vi "Spont7.vi"() -> ()   [LabVIEW 2014]
uses:
  <vilib>/Utility/file.llb/Write To Spreadsheet File (DBL).vi
panel:
  out "Identification":string
  out "Running":bool caption="C867_Multiaxis_Configuration_Setup.vi is running"
  out "Position":dbl[](array[numeric]) format="%.6f"
  in  "PI Stage Error":errorcluster
  out "GndNum":dbl
  out "Current Set":u32=24
  in  "time zero":dbl
  in  "Number of ground/series":dbl
  in  "Time points (fs)":dbl[](array[numeric])
  in  "Number of Series":dbl
  in  "take series":bool
  out "Status":string="Shutter Closed"
  in  "Shutter Position":bool
  in  "width":dbl=100.0
  in  "bottom row":dbl
  out "delta_counts":dbl=5.100000000000023
  out "cursor y":dbl=598.3
  out "Intensity Graph":u16[][](graph)
  in  "focus":bool
  in  "Filename":string="test"
  in  "SetPath":bool
  in  "Path":string="C:\\data"
  in  "Multi Acquire":bool
  in  "Number of acquisitions":dbl=10.0 format="%.3f"
  in  "Acquire":bool
  out "Temperature":dbl=-75.0
  in  "stop":bool
  in  "Save?":bool
  out "Waveform Graph":dbl[](graph)=[588.6, 596.72, 595.34, 596.64, 595.2, 596.1, 597.16, 596.12, 597.8, 597.66, 595.06, 597.86, 598.22, 596.64, 596.76, 597.44, 597.16, 596.86, 598.62, 597.82, 597.82, 598.04, 596.38, 597.32, 598.0, 596.96, 597.12, 596.68, 597.72, 595.7, 598.18, 596.84, 596.3, 596.74, 598.34, 595.84, 597.76, 597.96, 596.3, 597.2, 596.78, 595.68, 597.16, 597.9, 596.24, 596.52, 597.42, 596.5, 596.02, 596.42, 596.72, 595.96, 596.42, 596.8, 597.3, 594.68, 597.84, 596.16, 596.06, 595.2, 595.82, 595.88, 596.94, 596.26, 596.28, 595.88, 595.68, 596.14, 596.9, 597.08, 597.12, 596.2, 595.18, 595.26, 595.72, 596.18, 595.52, 595.84, 595.86, 596.56, 595.58, 596.64, 595.9, 596.54, 595.7, 595.56, 596.3, 596.8, 595.74, 596.68, 595.48, 596.96, 596.12, 595.02, 596.08, 595.96, 596.34, 596.14, 595.98, 595.84, 596.5, 595.88, 596.6, 595.96, 596.86, 596.28, 596.22, 595.8, 595.46, 596.18, 596.32, 596.0, 596.12, 596.22, 595.82, 595.76, 597.1, 596.46, 596.86, 596.48, 595.66, 595.94, 596.38, 595.46, 596.12, 596.36, 596.46, 596.7, 596.32, 596.84, 594.96, 595.22, 596.56, 596.52, 595.72, 596.22, 596.22, 596.38, 596.8, 595.52, 596.92, 597.12, 595.92, 596.18, 596.5, 597.3, 596.4, 596.46, 596.28, 597.04, 596.42, 595.84, 597.12, 596.66, 596.2, 597.02, 596.22, 596.12, 596.78, 595.68, 596.02, 595.36, 596.5, 596.9, 595.76, 595.12, 596.72, 597.54, 596.32, 596.76, 597.82, 597.52, 595.5, 595.88, 597.38, 596.3, 597.58, 595.42, 597.12, 597.58, 596.98, 597.44, 595.9, 596.58, 596.78, 597.04, 597.2, 596.06, 596.58, 597.08, 598.68, 596.32, 597.3, 597.28, 597.26, 595.9, 597.3, 597.98, 598.08, 598.16, 596.42, 597.82, 596.88, 597.34, 598.22, 598.38, 598.34, 597.66, 596.98, 597.18, 597.18, 597.7, 598.3, 597.3, 596.28, 597.0, 598.0, 598.42, 597.96, 596.32, 598.76, 597.32, 598.08, 598.1, 598.14, 598.06, 597.46, 598.08, 597.1, 597.88, 597.76, 598.74, 598.2, 598.54, 598.26, 596.74, 597.4, 597.82, 597.4, 597.64, 598.78, 597.84, 598.28, 596.68, 597.44, 598.66, 597.94, 598.2, 598.82, 598.28, 598.5, 597.86, 599.04, 597.96, 597.22, 598.38, 597.72, 598.18, 598.58, 598.44, 598.64, 598.98, 597.94, 598.84, 599.02, 598.76, 599.08, 599.0, 598.78, 597.5, 599.4, 598.52, 599.9, 597.04, 598.76, 598.3, 598.88, 599.76, 598.54, 599.92, 597.88, 598.42, 599.8, 599.8, 599.24, 598.58, 598.76, 597.02, 599.76, 599.84, 598.98, 599.5, 599.58, 599.46, 598.08, 599.3, 598.56, 598.74, 598.98, 598.74, 599.04, 599.18, 599.08, 598.64, 598.88, 599.04, 599.3, 598.54, 600.1, 599.12, 600.02, 599.32, 599.74, 600.04, 599.44, 598.96, 599.82, 601.1, 600.46, 599.48, 601.04, 599.16, 601.68, 600.5, 599.06, 599.0, 600.26, 600.54, 599.88, 599.62, 600.82, 601.56, 600.38, 600.6, 601.6, 599.1, 601.64, 600.56, 600.8, 601.94, 600.82, 599.68, 602.12, 602.36, 600.5, 601.56, 601.62, 601.04, 601.0, 602.0, 600.66, 601.34, 601.52, 600.86, 601.7, 600.28, 602.32, 602.78, 601.06, 600.34, 602.7, 602.52, 602.5, 601.3, 603.24, 601.06, 603.72, 603.78, 602.12, 601.68, 603.34, 602.0, 602.46, 602.64, 603.3, 601.6, 603.18, 603.1, 602.74, 602.32, 602.3, 603.38, 602.02, 602.82, 604.16, 603.64, 603.32, 603.84, 604.06, 603.82, 603.56, 602.68, 605.1, 602.58, 603.42, 603.36, 603.76, 602.68, 602.68, 602.22, 604.3, 602.44, 603.86, 603.74, 603.18, 603.32, 603.98, 604.28, 604.5, 602.92, 602.02, 604.08, 604.02, 604.02, 603.46, 603.42, 604.62, 602.96, 603.08, 604.44, 604.38, 603.66, 604.1, 603.98, 603.26, 603.46, 603.96, 604.54, 603.78, 603.98, 604.08, 604.18, 604.32, 605.34, 603.34, 605.42, 603.56, 604.22, 604.34, 604.32, 603.9, 603.66, 604.04, 605.02, 604.48, 604.16, 603.02, 603.8, 604.44, 604.66, 604.68, 604.12, 605.02, 604.86, 605.3, 604.54, 605.84, 604.78, 605.76, 604.86, 604.44, 605.16, 605.16, 604.86, 604.06, 605.46, 604.4, 603.62, 606.52, 606.38, 604.6, 605.34, 605.34, 604.98, 603.98, 605.5, 605.6, 604.54, 604.48, 604.3, 606.24, 605.36, 605.48, 605.36, 606.14, 605.26, 603.84, 604.94, 605.2, 605.16, 606.34, 604.56, 605.56, 605.74, 605.32, 605.34, 606.02, 607.14, 606.36, 605.08, 605.38, 606.54, 606.18, 607.14, 606.44, 606.22, 606.9, 606.66, 606.82, 606.76, 606.52, 606.24, 607.18, 606.6, 607.16, 609.14, 606.86, 606.68, 608.42, 606.66, 608.94, 608.54, 608.66, 608.4, 608.54, 608.54, 608.22, 608.26, 608.86, 608.4, 607.54, 607.48, 608.34, 610.3, 608.64, 607.96, 608.46, 609.12, 609.04, 607.74, 607.94, 609.82, 608.42, 609.24, 609.6, 608.64, 607.96, 608.92, 609.96, 609.78, 609.4, 608.54, 608.72, 607.38, 608.34, 609.22, 608.02, 608.38, 609.44, 608.12, 609.24, 609.06, 607.92, 609.1, 607.34, 609.76, 609.0, 609.04, 608.88, 607.82, 607.98, 608.34, 608.52, 609.72, 607.86, 608.1, 608.16, 607.1, 608.88, 606.4, 608.84, 608.48, 607.32, 608.34, 607.24, 608.02, 607.8, 608.04, 607.02, 608.8, 607.88, 608.4, 607.34, 607.66, 606.8, 607.2, 607.66, 608.94, 607.64, 608.6, 608.32, 607.64, 608.2, 608.02, 608.74, 607.9, 609.06, 606.98, 607.78, 607.6, 608.42, 607.68, 609.02, 608.2, 608.96, 607.76, 607.78, 608.84, 608.14, 609.02, 607.94, 608.8, 608.26, 608.9, 607.42, 608.9, 608.52, 607.1, 608.34, 608.44, 608.88, 608.28, 607.54, 607.88, 607.48, 608.28, 608.74, 608.64, 607.36, 608.72, 608.18, 608.5, 608.26, 609.14, 608.68, 608.34, 608.52, 608.24, 609.26, 609.5, 609.1, 607.4, 609.28, 609.72, 609.9, 609.22, 609.72, 609.66, 608.96, 609.84, 610.84, 610.26, 609.92, 609.36, 609.5, 609.14, 609.68, 609.52, 609.3, 608.82, 611.08, 610.52, 610.36, 610.02, 609.26, 609.7, 610.56, 609.24, 610.14, 609.78, 609.4, 611.1, 611.3, 611.64, 612.6, 610.7, 613.46, 611.62, 612.18, 610.72, 613.36, 612.92, 613.4, 612.44, 613.96, 612.2, 613.78, 615.38, 613.92, 613.36, 613.88, 615.7, 613.32, 613.66, 615.56, 615.4, 615.74, 616.56, 617.68, 614.58, 615.08, 616.86, 614.2, 615.56, 616.52, 616.36, 615.24, 616.04, 615.78, 615.56, 614.72, 616.18, 614.7, 614.36, 613.78, 614.8, 613.68, 614.04, 614.34, 613.14, 613.64, 613.64, 614.42, 612.28, 613.78, 612.32, 613.28, 611.98, 613.0, 612.32, 611.54, 612.3, 612.14, 610.24, 611.56, 611.84, 609.42, 610.02, 608.86, 609.02, 608.0, 609.18, 608.92, 608.78, 608.16, 608.16, 607.16, 607.6, 605.94, 607.6, 607.18, 607.04, 607.18, 605.5, 607.02, 605.26, 604.78, 606.2, 605.3, 604.52, 604.9, 604.58, 603.74, 604.46, 605.02, 603.8, 604.58, 603.5, 603.18, 603.26, 603.48, 603.56, 604.36, 602.92, 602.44, 603.58, 604.18, 603.16, 602.2, 603.7, 603.12, 602.68, 601.74, 602.14, 602.48, 602.62, 602.0, 602.22, 602.06, 600.94, 601.92, 601.28, 602.22, 601.72, 601.44, 602.04, 603.22, 601.52, 601.36, 602.06, 601.96, 602.14, 601.68, 601.28, 602.46, 601.56, 601.44, 602.1, 602.1, 601.8, 603.02, 601.12, 599.86, 601.56, 600.46, 601.28, 601.18, 600.58, 599.68, 600.74, 600.74, 601.66, 600.72, 600.6, 602.3, 599.66, 601.5, 602.32, 601.38, 600.18, 600.76, 601.32, 599.64, 601.16, 599.82, 600.52, 600.66, 601.66, 600.36, 600.18, 599.8, 601.42, 601.12, 599.68, 600.6, 600.42, 599.92, 600.98, 600.56, 599.54, 600.46, 601.52, 601.1, 599.78, 600.84, 599.98, 600.6, 599.16, 599.74, 600.46, 600.42, 600.62, 599.84, 599.66, 600.98, 600.98, 600.94, 601.16, 602.18, 601.28, 600.56, 601.56, 600.94, 602.32, 600.34, 601.98, 602.02, 601.46, 602.86, 603.68, 603.04, 601.86, 602.02, 601.94, 602.36, 601.96, 602.14, 602.42, 603.9, 602.9, 602.66, 602.48, 603.4, 603.32, 601.5, 603.14, 601.3, 601.94, 603.14, 602.58, 601.6, 600.16, 602.08, 600.76, 599.68, 602.42, 601.32, 600.14, 600.22, 599.8, 600.3, 598.68, 599.82, 599.72, 599.24, 599.36, 599.64, 599.34, 598.94, 598.82, 598.82, 597.72, 599.52, 598.6, 598.18, 597.34, 598.04, 597.26, 598.3, 598.18, 597.88, 596.96, 598.36, 597.14, 597.7, 597.7, 598.32, 597.54, 598.62, 596.16, 598.24, 598.36, 596.74, 597.62, 597.46, 596.92, 597.18, 598.18, 597.04, 596.94, 596.78, 596.92, 597.72, 596.84, 596.98, 597.02, 597.44, 597.34, 597.98, 596.28, 598.24, 597.62, 596.52, 596.6, 597.32, 596.58, 597.78, 597.82, 596.64, 596.28, 597.64, 597.14, 597.4, 597.42, 597.6, 596.1, 597.04, 597.94, 597.38, 597.08, 597.4, 597.66, 596.64, 597.68, 597.6, 596.6, 598.68, 597.3, 596.06, 596.9, 596.22, 597.14, 596.6, 597.3, 596.32, 596.6, 596.8, 595.5, 597.28, 597.02, 596.42, 596.58, 595.22, 596.26, 597.54, 597.24, 597.04, 596.62, 597.18, 596.72, 596.56, 596.82, 596.96, 595.0, 595.9, 596.66, 596.98, 595.36, 595.84, 596.92, 596.84, 596.5, 598.1, 595.56, 596.7, 596.2, 596.66, 595.92, 597.0, 596.86, 595.82, 596.24, 596.7, 596.66, 596.36, 597.12, 597.48, 596.52, 598.24, 596.88, 596.66, 596.18, 597.32, 596.68, 596.6, 597.56, 597.46, 597.28, 596.44, 598.22, 596.78, 597.58, 596.9, 597.02, 597.7, 598.36, 597.7, 597.82, 597.6, 596.76, 598.34, 596.64, 597.76, 597.26, 597.26, 597.2, 598.16, 598.38, 596.48, 597.54, 598.78, 597.72, 597.6, 596.28, 597.92, 596.92, 597.46, 597.82, 597.7, 596.92, 598.0, 598.34, 598.0, 598.1, 596.42, 597.68, 597.0, 597.04, 598.34, 598.08, 598.16, 597.44, 596.68, 598.76, 598.98, 597.34, 598.54, 597.74, 598.16, 597.02, 597.82, 596.48, 599.84, 598.26, 599.96, 598.18, 598.06, 596.84, 597.94, 597.86, 597.82, 597.2, 597.74, 598.74, 598.66, 599.84, 599.12, 599.16, 598.22, 599.14, 598.3, 599.32, 599.28, 598.04, 599.02, 600.24, 598.9, 598.52, 600.26, 599.12, 599.52, 600.16, 598.7, 600.54, 600.4, 600.34, 599.94, 601.08, 601.94, 601.8, 601.84, 600.94, 602.66, 602.7, 603.24, 603.4, 603.48, 603.54, 604.46, 603.48, 604.86, 604.02, 605.42, 605.5, 605.6, 605.66, 606.92, 606.64, 607.8, 608.02, 606.8, 607.34, 608.3, 608.7, 609.58, 607.02, 608.78, 609.04, 608.58, 608.68, 607.9, 607.96, 608.04, 606.88, 607.1, 608.22, 606.34, 606.48, 605.72, 607.14, 607.1, 606.26, 605.84, 605.2, 606.94, 605.42, 605.78, 604.82, 604.0, 604.46, 604.06, 604.12, 604.18, 602.44, 602.64, 602.74, 602.96, 602.62, 602.58, 601.22, 601.08, 601.62, 601.8, 600.3, 600.86, 600.84, 601.36, 601.52, 600.26, 601.46, 601.82, 601.08, 601.38, 600.68, 601.24, 600.14, 600.86, 601.44, 601.02, 601.64, 600.2, 600.14, 600.08, 601.2, 600.78, 600.14, 600.7, 600.84, 600.46, 600.52, 601.54, 600.18, 601.48, 601.34, 600.8, 600.14, 600.98, 601.96, 601.24, 599.72, 601.54, 601.0, 601.22, 602.3, 601.8, 600.8, 602.04, 601.66, 602.18, 602.98, 601.9, 600.84, 601.02, 602.26, 602.6, 601.68, 602.74, 603.4, 603.34, 601.14, 603.26, 603.8, 602.5, 605.12, 607.2, 608.98, 613.54, 618.18, 624.58, 630.92, 637.18, 645.2, 652.4, 662.02, 675.08, 685.88, 712.56, 745.04, 764.62, 788.84, 800.84, 817.9, 850.88, 881.62, 935.36, 970.52, 991.22, 1024.2, 1039.16, 1063.5, 1047.88, 1030.98, 1037.14, 1049.92, 1025.08, 960.02, 939.14, 920.52, 907.38, 895.3, 884.3, 860.94, 811.92, 782.22, 752.82, 733.08, 720.42, 706.32, 693.9, 683.38, 676.24, 667.8, 659.5, 652.08, 648.94, 646.08, 642.08, 637.86, 633.48, 631.2, 628.9, 626.92, 625.0, 622.5, 622.22, 619.52, 621.44, 618.92, 619.38, 619.44]
  in  "Exposure Time (s)":dbl=20.0 format="%.3f"
  out "error out":errorcluster
  in  "error in (no error)":errorcluster
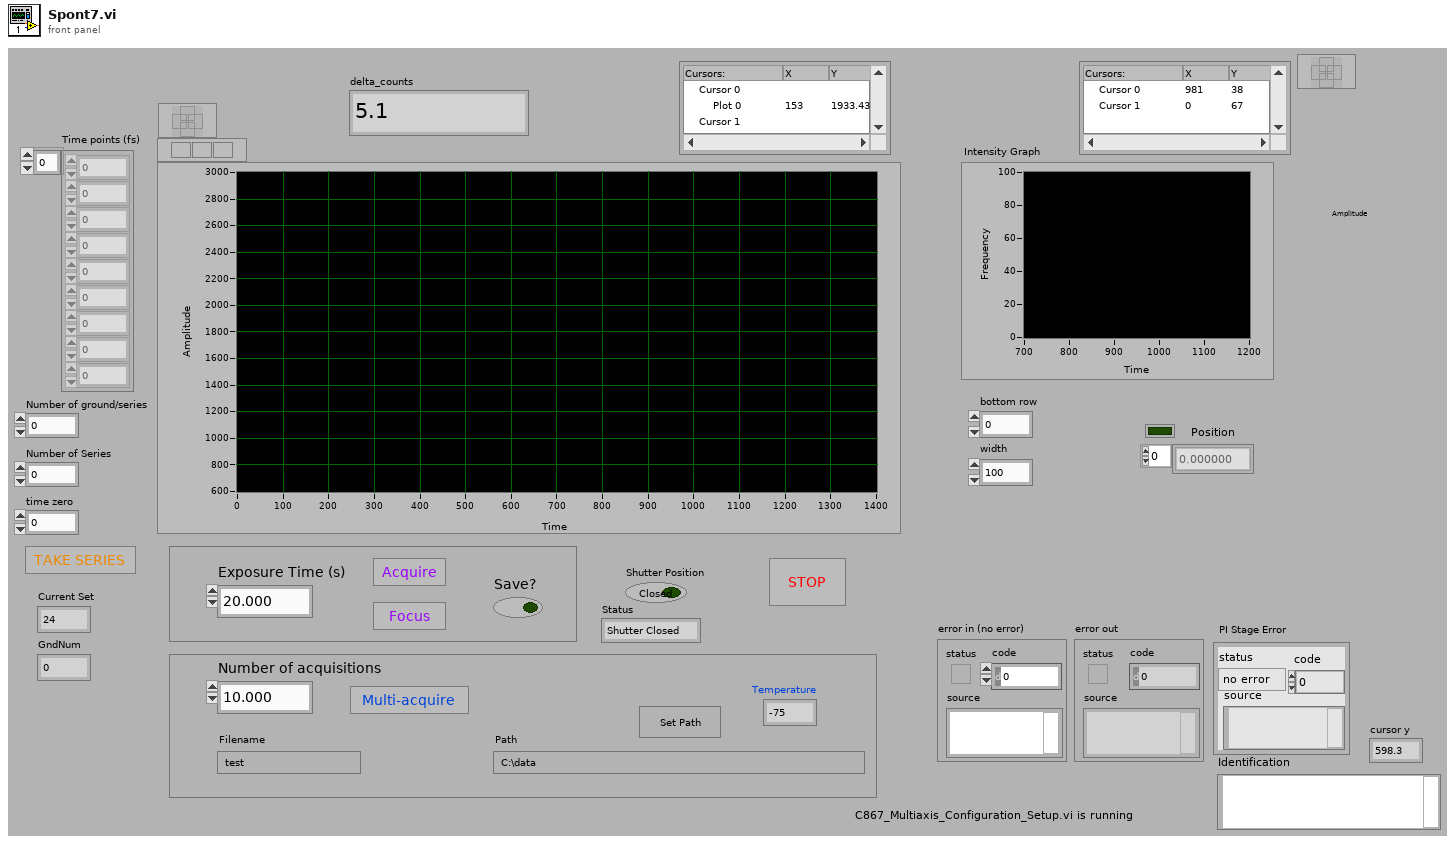
[diagram p1: front panel]
types:
  T1 = cluster{"Camera Handle":u32, "File Handle":u32, "Image Handle":u32}
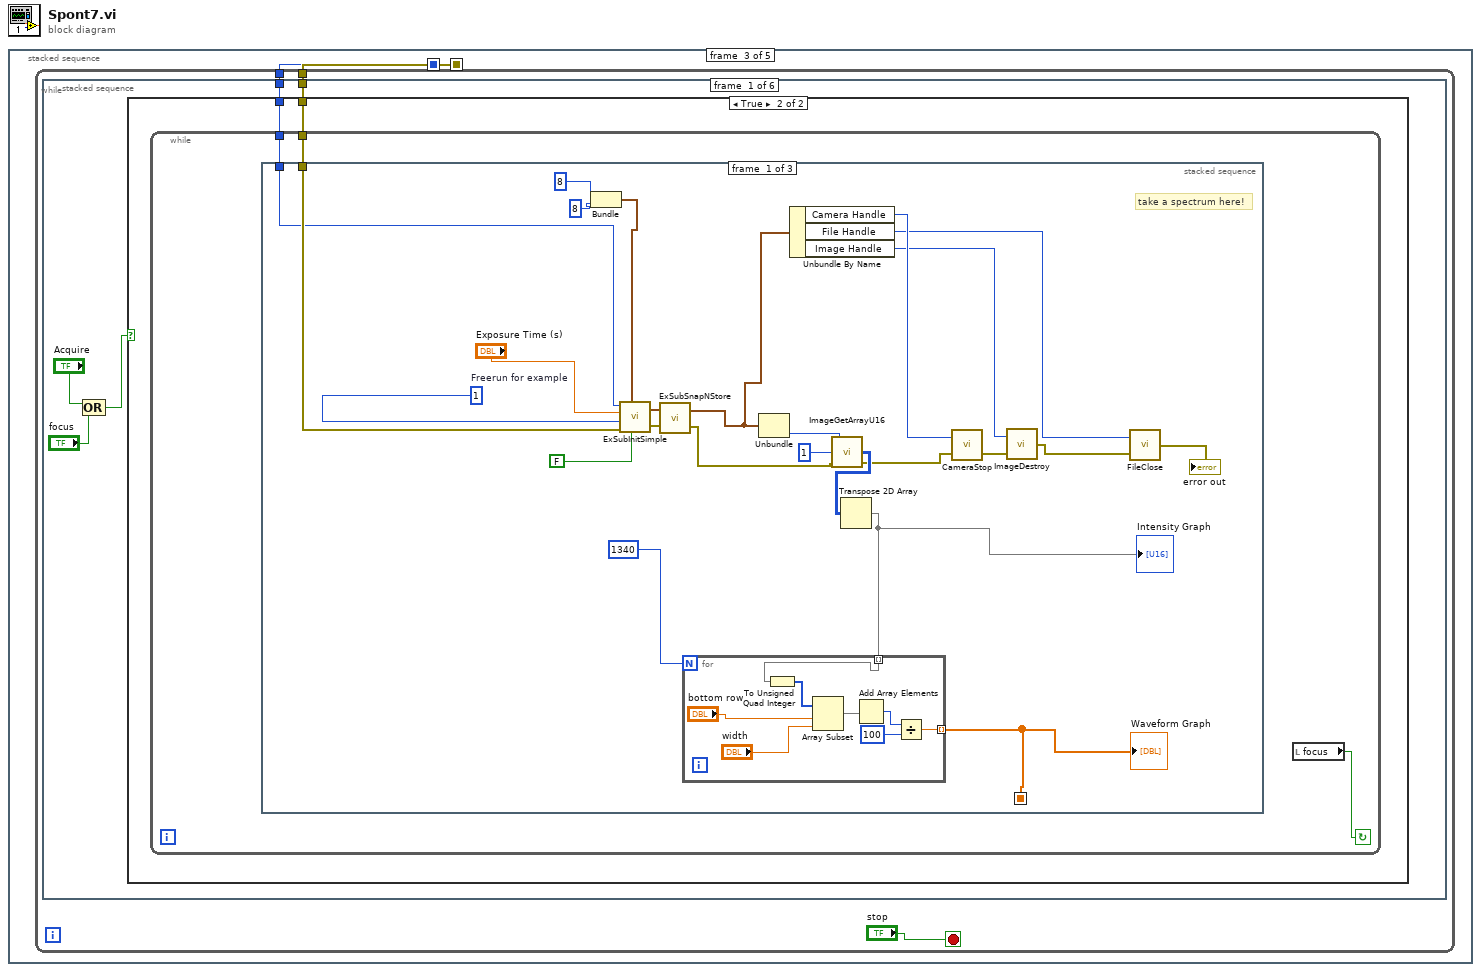
[diagram p0: block diagram]
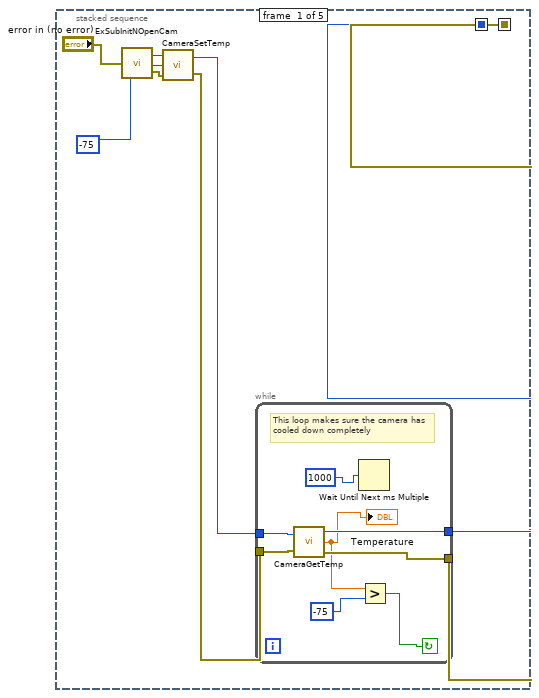
[diagram p2: hidden frame]
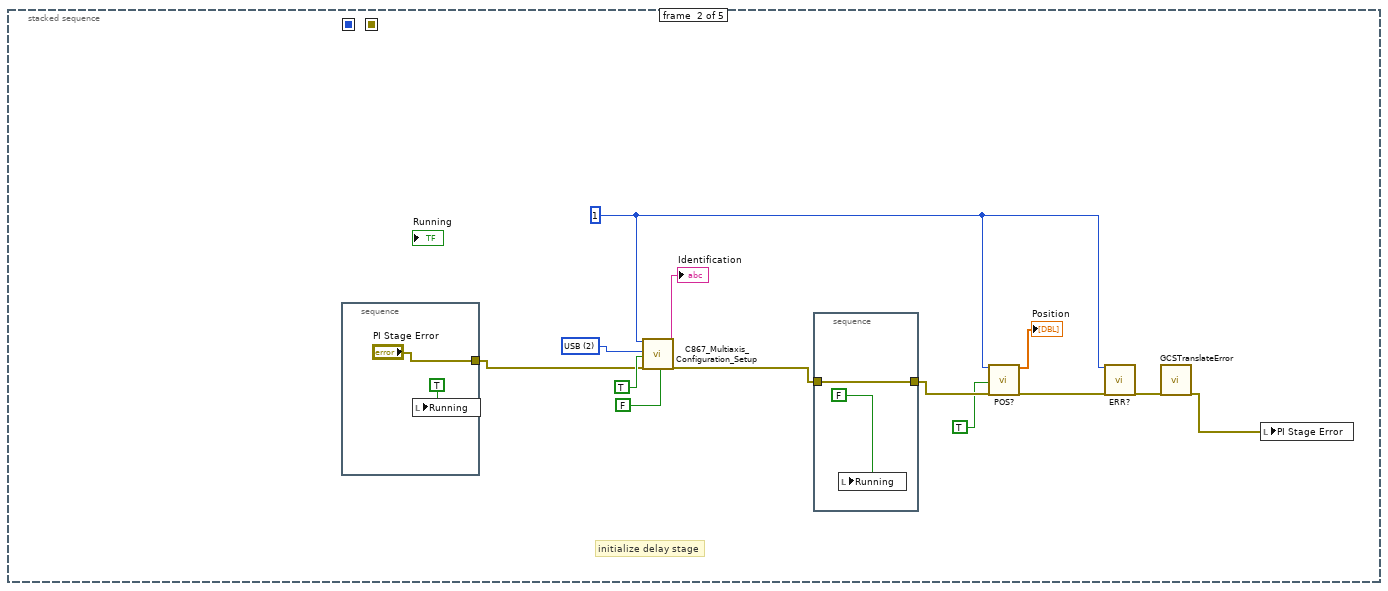
[diagram p3: hidden frame]
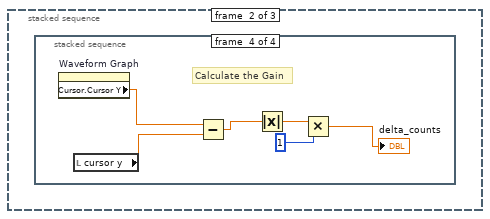
[diagram p5: hidden frame]
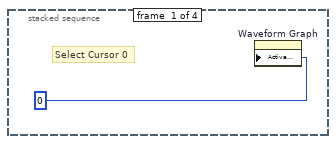
[diagram p6: hidden frame]
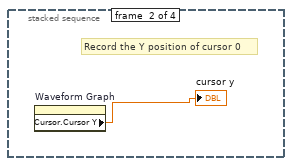
[diagram p7: hidden frame]
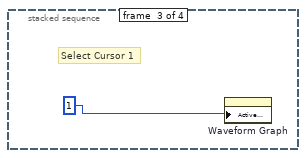
[diagram p8: hidden frame]
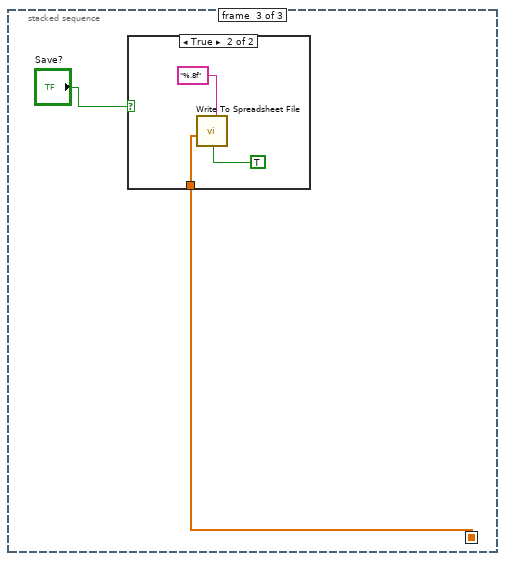
[diagram p9: hidden frame]
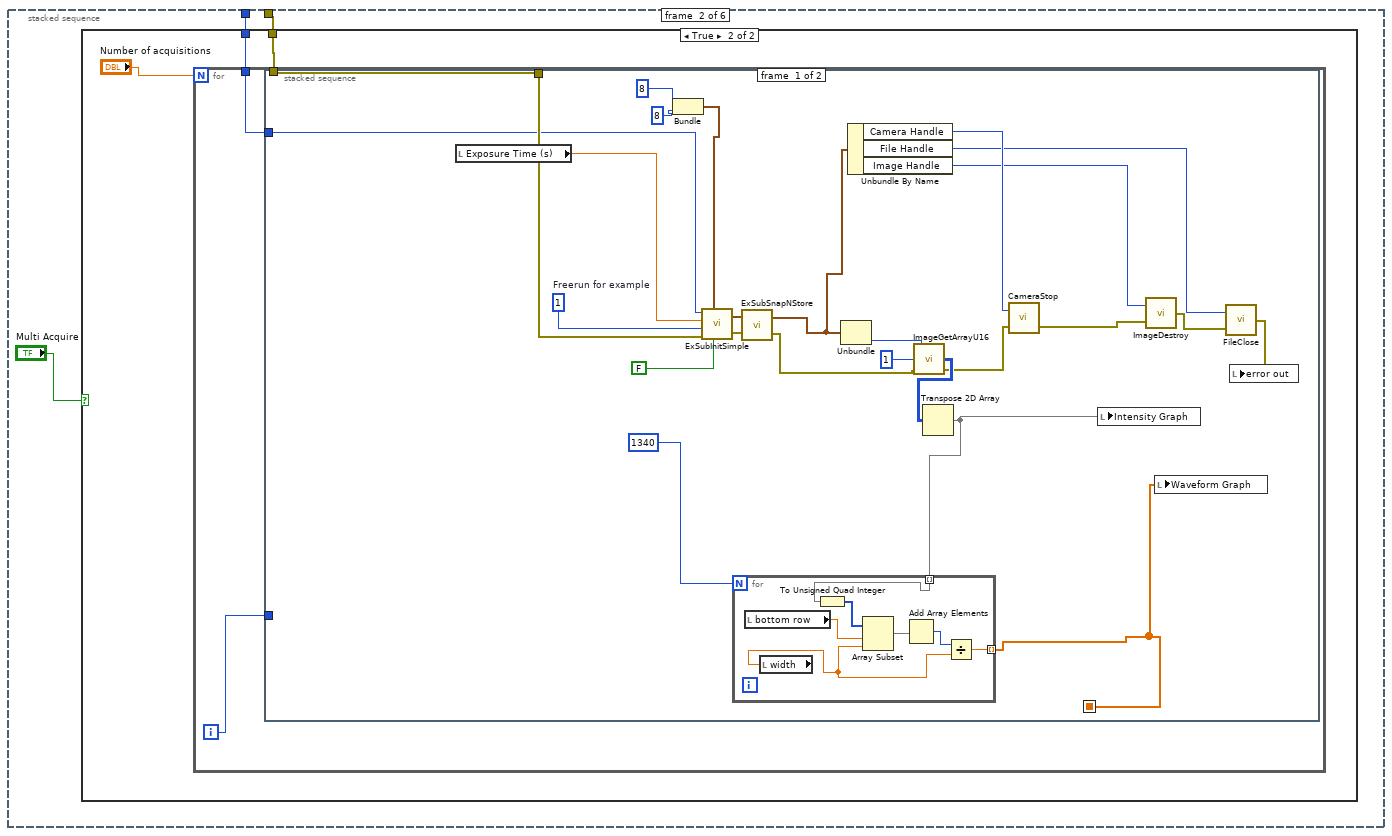
[diagram p11: hidden frame]
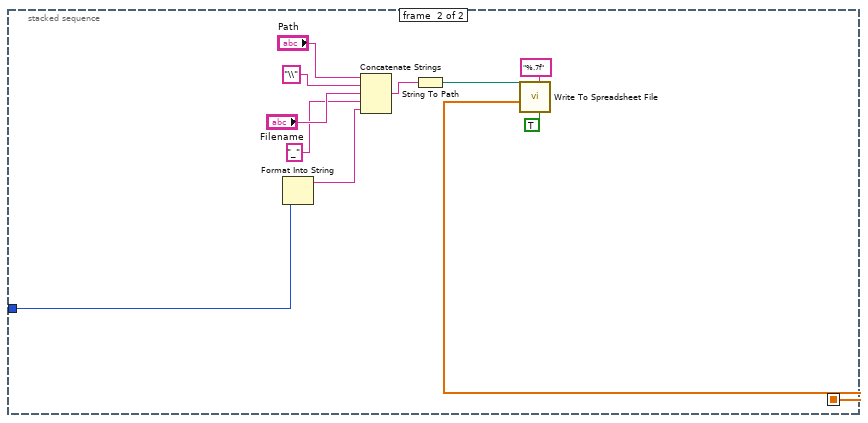
[diagram p13: hidden frame]
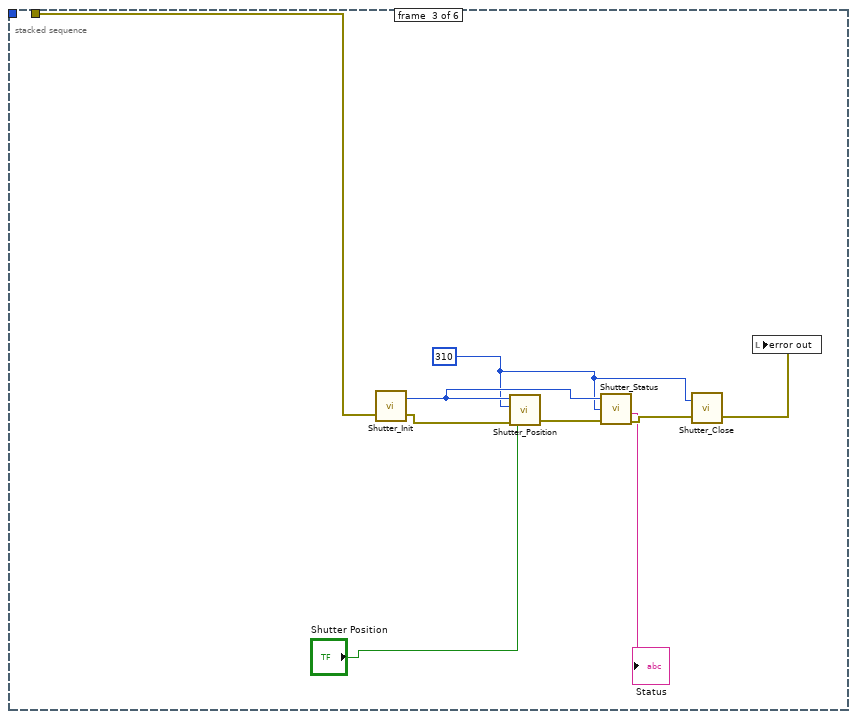
[diagram p14: hidden frame]
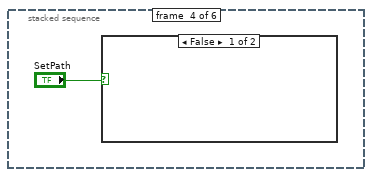
[diagram p15: hidden frame]
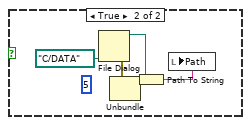
[diagram p16: hidden frame]
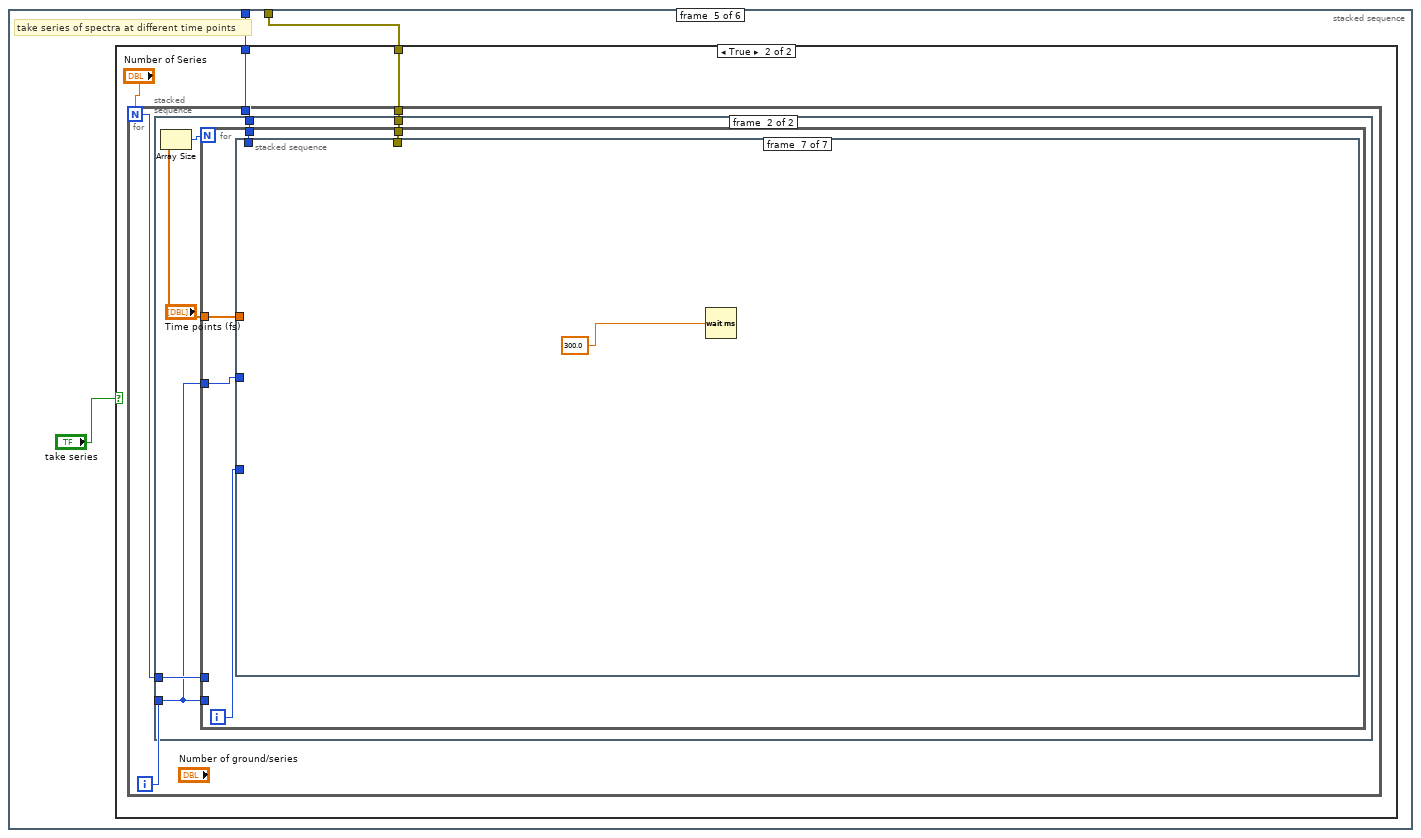
[diagram p17: hidden frame]
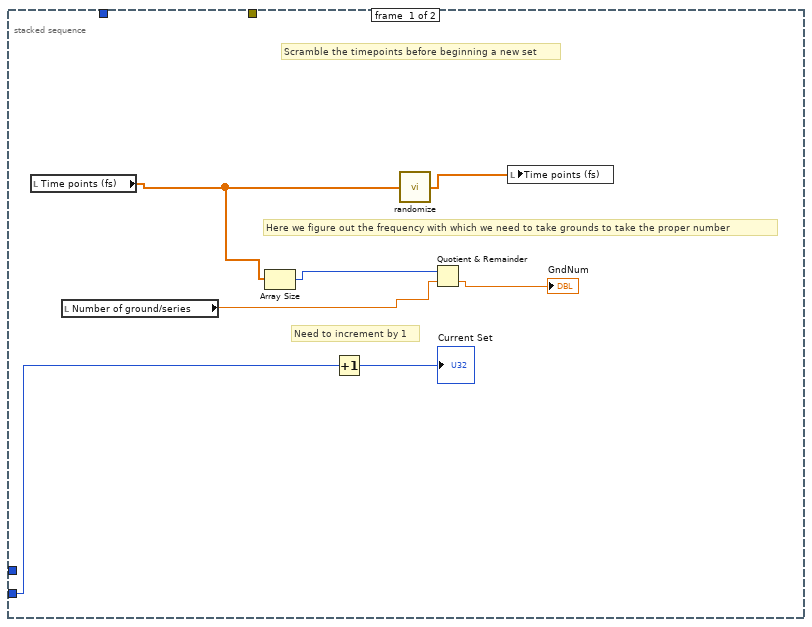
[diagram p19: hidden frame]
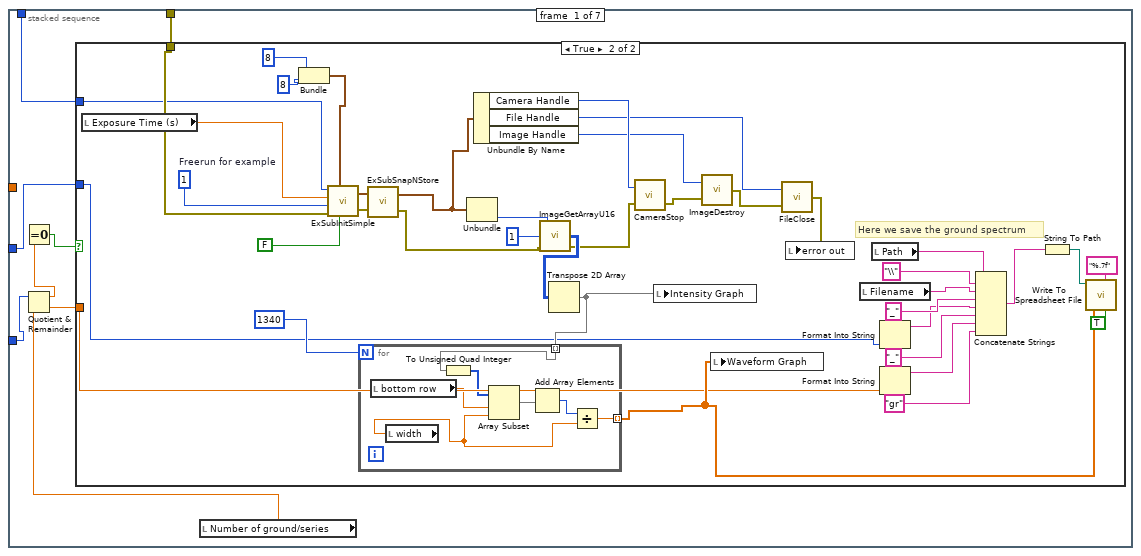
[diagram p20: hidden frame]
diagram:
  n1 = stacked-sequence {
    seq-local: [w2 _ _ _ _] -> [_ _ w35 _ w325]
    seq-local: [w1 _ _ _ _] -> [_ _ w34 _ w326]
    frame #0 {
      n2 = call "ExSubInitNOpenCam.vi"("error in (no error)"="error in (no error)") -> ("Camera Handle"=w5:u32, "error out"=w7:errorcluster)
      n3 = call <userlib>:"CameraSetTemp.vi"("error in (no error)"=w7, "Temperature"=-75, "Camera Handle"=w5) -> ("error out"=w3:errorcluster, "Camera Handle"=w4:u32)
      n4 = while {
        tunnel: w3 -> [w15]
        tunnel: [w14] -> w2
        tunnel: w4 -> [w13]
        tunnel: [w12] -> w1
        stop <- w10 continue-if-true
        # "This loop makes sure the camera has cooled down completely"
        n5 = call <userlib>:"CameraGetTemp.vi"("Camera Handle"=w13, "error in (no error)"=w15) -> ("Camera Handle"=w12:u32, "Temperature"=w9:dbl, "error out"=w14:errorcluster)
        "Temperature" <- w9
        n6 = Wait Until Next ms Multiple(millisecond multiple=1000 ("ADC Gain")) -> ()  [unwired: 1 out]
        n7 = Greater?(x=w9, y=-75) -> (0:w10:bool)
      }
    }
    frame #1 {
      w20 = 1 ("System no.")
      w29 = u16 2 items=["RS232", "RS232 DaisyChain", "USB"] ("Interface")
      # "initialize delay stage"
      n8 = stacked-sequence {
        tunnel: ["PI Stage Error"] -> w26
        frame #0 {
          n9 = local write "Running"(TRUE ("Running")) -> ()
        }
      }
      n10 = call "C867_Multiaxis_Configuration_Setup.vi"("System no."=w20, "Interface"=w29, "All axes?"=TRUE, "error in"=w26, "Switch servo on?"=FALSE ("Use dialog to define\nconnected stages?")) -> ("Identification"=→"Identification":string, "error out"=w25:errorcluster)  [unwired: 8 in, 5 out]
      n11 = stacked-sequence {
        tunnel: w25 -> [w31]
        tunnel: [w31] -> w23
        frame #0 {
          n12 = local write "Running"(FALSE ("Running")) -> ()
        }
      }
      n13 = call "POS?.vi"("System no."=w20, "All axes?"=TRUE, "error in"=w23) -> ("Position"=→"Position":dbl[], "error out"=w21:errorcluster)  [unwired: 15 in]
      n14 = call "ERR?.vi"("System no."=w20, "error in"=w21) -> ("error out"=w19:errorcluster)  [unwired: 16 in, 1 out]
      n15 = call "GCSTranslateError.vi"("error in"=w19) -> ("error out"=w17:errorcluster)  [unwired: 16 in, 2 out]
      n16 = local write "PI Stage Error"(w17) -> ()
    }
    frame #2 {
      n17 = while {
        tunnel: w35 -> [w37]
        tunnel: w34 -> [w36]
        stop <- "stop" stop-if-true
        n18 = stacked-sequence {
          tunnel: w37 -> [w43 w97 w149 _ w163 _]
          tunnel: w36 -> [w42 w96 _ _ w162 _]
          frame #0 {
            n19 = Compound Arithmetic op=OR("Acquire", "focus") -> (w39:bool)
            n20 = case shown="True" w39 {
              tunnel: w43 -> [_ w45]
              tunnel: w42 -> [_ w44]
              frame False {
              }
              frame True {
                n21 = while {
                  tunnel: w45 -> [w48]
                  tunnel: w44 -> [w47]
                  stop <- w46 continue-if-true
                  n22 = stacked-sequence {
                    seq-local: [w60 _ _] -> [_ _ w91]
                    tunnel: w48 -> [w59 _ _]
                    tunnel: w47 -> [w58 _ _]
                    frame #0 {
                      w71 = 1  # Freerun for example
                      # "take a spectrum here!"
                      n23 = Bundle(8, 8) -> (w69:cluster{i32, i32})  [unwired: 1 in]
                      n24 = call "ExSubInitSimple.vi"("Intensifier"=FALSE, "Shutter Comp"=w69, "error in (no error)"=w59, "Triggering mode"=w71, "Exposure"="Exposure Time (s)", "Camera Handle"=w58) -> ("error out"=w68:errorcluster, "Handles"=w67:cluster{"Camera":u32, "File":u32, "Image":u32})
                      n25 = call "ExSubSnapNStore.vi"("error in (no error)"=w68, "Handle Cluster"=w67) -> ("error out"=w63:errorcluster, "Handle Cluster Out"=w57:T1)
                      n26 = Unbundle(w57) -> ("Image Handle"=w64:u32)  [unwired: 2 out]
                      n27 = Unbundle By Name(w57) -> ("Camera Handle"=w56:u32, "File Handle"=w55:u32, "Image Handle"=w52:u32)
                      n28 = call <userlib>:"ImageGetArrayU16.vi"("error in"=w63, "Z position"=1, "Image Handle"=w64) -> ("error out"=w54:errorcluster, "Array uint 16"=w62:u16[][])  [unwired: 1 out]
                      n29 = Transpose 2D Array(2D array=w62) -> (transposed array=w49:u16[][])
                      "Intensity Graph" <- w49
                      n30 = for {
                        N: 1340 -> [_]
                        tunnel: w49 -> [w78] mode=indexing
                        tunnel: [w80] -> w60 mode=indexing
                        n31 = To Unsigned Quad Integer(1:w78) -> (0:w77:u64[])
                        n32 = Array Subset(array=w77, index="bottom row", length="width") -> (w79:u64[])
                        n33 = Add Array Elements(numeric array=w79) -> (sum=w81:u64)
                        n34 = Divide(x=w81, y=u64 100) -> (x/y=w80:dbl)
                      }
                      "Waveform Graph" <- w60
                      n35 = call <userlib>:"CameraStop.vi"("error in"=w54, "Camera Handle"=w56) -> ("error out"=w51:errorcluster)  [unwired: 1 out]
                      n36 = call <userlib>:"ImageDestroy.vi"("error in"=w51, "Data handle"=w52) -> ("error out"=w50:errorcluster)
                      n37 = call <userlib>:"FileClose.vi"("error in"=w50, "File Handle"=w55) -> ("error out"=→"error out":errorcluster)
                    }
                    frame #1 {
                      n38 = stacked-sequence {
                        frame #0 {
                          # "Select Cursor 0"
                          n39 = property on="Waveform Graph" class="WFGraph (strict)"("Active Cursor"=0) -> ()  [unwired: 2 in, 2 out]
                        }
                        frame #1 {
                          # "Record the Y position of cursor 0"
                          n40 = property on="Waveform Graph" class="WFGraph (strict)"() -> ("Cursor.Cursor Y"=→"cursor y":dbl)  [unwired: 2 in, 2 out]
                        }
                        frame #2 {
                          # "Select Cursor 1"
                          n41 = property on="Waveform Graph" class="WFGraph (strict)"("Active Cursor"=1) -> ()  [unwired: 2 in, 2 out]
                        }
                        frame #3 {
                          # "Calculate the Gain"
                          n42 = property on="Waveform Graph" class="WFGraph (strict)"() -> ("Cursor.Cursor Y"=w85:dbl)  [unwired: 2 in, 2 out]
                          n43 = local read "cursor y"() -> (w90:dbl)
                          n44 = Subtract(x=w85, y=w90) -> (x-y=w87:dbl)
                          n45 = Absolute Value(x=w87) -> (abs(x)=w89:dbl)
                          n46 = Multiply(x=w89, y=1) -> (x*y=→"delta_counts":dbl)
                        }
                      }
                    }
                    frame #2 {
                      n47 = case shown="True" "Save?" {
                        tunnel: w91 -> [_ w94]
                        frame False {
                        }
                        frame True {
                          n48 = call-poly <vilib>:"Write To Spreadsheet File.vi"("transpose? (no:F)"=TRUE, "format (%.3f)"="%.8f", "1D data"=w94) -> ()  [unwired: 5 in, 1 out]
                        }
                      }
                    }
                  }
                  n49 = local read "focus"() -> (w46:bool)
                }
              }
            }
          }
          frame #1 {
            n50 = case shown="True" "Multi Acquire" {
              tunnel: w97 -> [_ w100]
              tunnel: w96 -> [_ w99]
              frame False {
              }
              frame True {
                n51 = for {
                  N: "Number of acquisitions" -> [_]
                  tunnel: w100 -> [w103]
                  tunnel: w99 -> [w102]
                  i -> [w104]
                  n52 = stacked-sequence {
                    seq-local: [w106 _] -> [_ w137]
                    tunnel: w104 -> [_ w147]
                    tunnel: w103 -> [w118 _]
                    tunnel: w102 -> [w117 _]
                    frame #0 {
                      w127 = 1  # Freerun for example
                      n53 = local read "Exposure Time (s)"() -> (w116:dbl)
                      n54 = Bundle(8, 8) -> (w126:cluster{i32, i32})  [unwired: 1 in]
                      n55 = call "ExSubInitSimple.vi"("Intensifier"=FALSE, "Shutter Comp"=w126, "error in (no error)"=w118, "Triggering mode"=w127, "Exposure"=w116, "Camera Handle"=w117) -> ("error out"=w125:errorcluster, "Handles"=w124:cluster{"Camera":u32, "File":u32, "Image":u32})
                      n56 = call "ExSubSnapNStore.vi"("error in (no error)"=w125, "Handle Cluster"=w124) -> ("error out"=w120:errorcluster, "Handle Cluster Out"=w113:T1)
                      n57 = Unbundle(w113) -> ("Image Handle"=w121:u32)  [unwired: 2 out]
                      n58 = Unbundle By Name(w113) -> ("Camera Handle"=w115:u32, "File Handle"=w114:u32, "Image Handle"=w109:u32)
                      n59 = call <userlib>:"ImageGetArrayU16.vi"("error in"=w120, "Z position"=1, "Image Handle"=w121) -> ("error out"=w112:errorcluster, "Array uint 16"=w119:u16[][])  [unwired: 1 out]
                      n60 = Transpose 2D Array(2D array=w119) -> (transposed array=w105:u16[][])
                      n61 = for {
                        N: 1340 -> [_]
                        tunnel: w105 -> [w133] mode=indexing
                        tunnel: [w135] -> w106 mode=indexing
                        n62 = local read "bottom row"() -> (w131:dbl)
                        n63 = local read "width"() -> (w130:dbl)
                        n64 = To Unsigned Quad Integer(1:w133) -> (0:w132:u64[])
                        n65 = Array Subset(array=w132, index=w131, length=w130) -> (w134:u64[])
                        n66 = Add Array Elements(numeric array=w134) -> (sum=w136:u64)
                        n67 = Divide(x=w136, y=w130) -> (x/y=w135:dbl)
                      }
                      n68 = call <userlib>:"CameraStop.vi"("error in"=w112, "Camera Handle"=w115) -> ("error out"=w110:errorcluster)  [unwired: 1 out]
                      n69 = local write "Intensity Graph"(w105) -> ()
                      n70 = call <userlib>:"ImageDestroy.vi"("error in"=w110, "Data handle"=w109) -> ("error out"=w108:errorcluster)
                      n71 = local write "Waveform Graph"(w106) -> ()
                      n72 = call <userlib>:"FileClose.vi"("error in"=w108, "File Handle"=w114) -> ("error out"=w111:errorcluster)
                      n73 = local write "error out"(w111) -> ()
                    }
                    frame #1 {
                      n74 = Format Into String(w147) -> (resulting string=w142:string)  [unwired: 3 in, 1 out]
                      n75 = Concatenate Strings("Path", "\\", "Filename", "_", w142) -> (w141:string)
                      n76 = String To Path(string=w141) -> (path=w138:path)
                      n77 = call-poly <vilib>:"Write To Spreadsheet File.vi"("transpose? (no:F)"=TRUE, "format (%.3f)"="%.7f", "1D data"=w137, "file path (dialog if empty)"=w138) -> ()  [unwired: 4 in, 1 out]
                    }
                  }
                }
              }
            }
          }
          frame #2 {
            w151 = 310
            n78 = call "Shutter_Init.vi"("error in"=w149) -> ("error out"=w156:errorcluster, "ObjectPtr"=w153:i32)  [unwired: 1 in]
            n79 = call "Shutter_Position.vi"("error in"=w156, "Shutter Position"="Shutter Position", "ShutterID"=w151, "ObjectPtr"=w153) -> ("error out"=w155:errorcluster)  [unwired: 2 in]
            n80 = call "Shutter_Status.vi"("ObjectPtr"=w153, "ShutterID"=w151, "error in"=w155) -> ("Status"=→"Status":string, "error out"=w154:errorcluster)  [unwired: 2 out]
            n81 = call "Shutter_Close.vi"("error in"=w154, "ObjectPtr"=w151) -> ("error out"=w148:errorcluster)  [unwired: 1 in]
            n82 = local write "error out"(w148) -> ()
          }
          frame #3 {
            n83 = case shown="False" "SetPath" {
              frame False {
              }
              frame True {
                (unwired) 5
                n84 = File Dialog(11:path "C:/DATA") -> (0:w158:errorcluster, 3:w161:path)  [unwired: 6 in, 2 out]
                n85 = Unbundle(w158) -> ()  [unwired: 3 out]
                n86 = Path To String(path=w161) -> (string=w159:string)
                n87 = local write "Path"(w159) -> ()
              }
            }
          }
          frame #4 {
            # "take series of spectra at different time points"
            n88 = case shown="True" "take series" {
              tunnel: w163 -> [_ w166]
              tunnel: w162 -> [_ w165]
              frame False {
              }
              frame True {
                n89 = for {
                  N: "Number of Series" -> [w171]
                  tunnel: w166 -> [w169]
                  tunnel: w165 -> [w168]
                  i -> [w170]
                  n90 = stacked-sequence {
                    tunnel: w171 -> [_ w182]
                    tunnel: w170 -> [w175 w181]
                    tunnel: w169 -> [_ w180]
                    tunnel: w168 -> [_ w179]
                    frame #0 {
                      # "Here we figure out the frequency with which we need to take grounds to take the proper number"
                      # "Need to increment by 1"
                      # "Scramble the timepoints before beginning a new set"
                      n91 = local read "Time points (fs)"() -> (w173:dbl[])
                      n92 = local read "Number of ground/series"() -> (w177:dbl)
                      n93 = Array Size(array=w173) -> (size(s)=w172:i32)
                      n94 = Increment(x=w175) -> (x+1=→"Current Set":i32)
                      n95 = call "randomize.vi"("Input array"=w173) -> ("Output array"=w176:dbl[])
                      n96 = Quotient & Remainder(x=w172, y=w177) -> (floor(x/y)=→"GndNum":dbl)  [unwired: 1 out]
                      n97 = local write "Time points (fs)"(w176) -> ()
                    }
                    frame #1 {
                      n98 = Array Size(array="Time points (fs)") -> (size(s)=w184:i32)
                      n99 = for {
                        N: w184 -> [_]
                        tunnel: "Time points (fs)" -> [w187]
                        tunnel: w181 -> [_]
                        tunnel: w182 -> [_]
                        tunnel: w181 -> [w189]
                        tunnel: w180 -> [w186]
                        tunnel: w179 -> [w185]
                        i -> [w188]
                        n100 = stacked-sequence {
                          tunnel: w189 -> [w193 _ _ w264 _ _ _]
                          tunnel: w188 -> [w195 w244 _ w265 _ _ _]
                          tunnel: w187 -> [_ w245 _ w266 _ _ _]
                          tunnel: w186 -> [w191 _ w259 w280 w312 _ _]
                          tunnel: w185 -> [w190 _ _ _ _ _ _]
                          frame #0 {
                            n101 = local read "Number of ground/series"() -> (w196:dbl)
                            n102 = Quotient & Remainder(x=w195, y=w196) -> (x-y*floor(x/y)=w197:dbl, floor(x/y)=w192:dbl)
                            n103 = Equal To 0?(x=w197) -> (x = 0?=w194:bool)
                            n104 = case shown="True" w194 {
                              tunnel: w193 -> [_ w198]
                              tunnel: w192 -> [_ w199]
                              tunnel: w191 -> [_ w236]
                              tunnel: w190 -> [_ w235]
                              frame False {
                              }
                              frame True {
                                w233 = 1  # Freerun for example
                                # "Here we save the ground spectrum"
                                n105 = local read "Exposure Time (s)"() -> (w224:dbl)
                                n106 = Bundle(8, 8) -> (w232:cluster{i32, i32})  [unwired: 1 in]
                                n107 = call "ExSubInitSimple.vi"("Intensifier"=FALSE, "Shutter Comp"=w232, "error in (no error)"=w236, "Triggering mode"=w233, "Exposure"=w224, "Camera Handle"=w235) -> ("error out"=w231:errorcluster, "Handles"=w230:cluster{"Camera":u32, "File":u32, "Image":u32})
                                n108 = call "ExSubSnapNStore.vi"("error in (no error)"=w231, "Handle Cluster"=w230) -> ("error out"=w226:errorcluster, "Handle Cluster Out"=w221:T1)
                                n109 = Unbundle(w221) -> ("Image Handle"=w227:u32)  [unwired: 2 out]
                                n110 = Unbundle By Name(w221) -> ("Camera Handle"=w223:u32, "File Handle"=w222:u32, "Image Handle"=w217:u32)
                                n111 = call <userlib>:"ImageGetArrayU16.vi"("error in"=w226, "Z position"=1, "Image Handle"=w227) -> ("error out"=w220:errorcluster, "Array uint 16"=w225:u16[][])  [unwired: 1 out]
                                n112 = Transpose 2D Array(2D array=w225) -> (transposed array=w214:u16[][])
                                n113 = for {
                                N: 1340 -> [_]
                                tunnel: w214 -> [w240] mode=indexing
                                tunnel: [w242] -> w200 mode=indexing
                                n114 = local read "bottom row"() -> (w238:dbl)
                                n115 = local read "width"() -> (w237:dbl)
                                n116 = To Unsigned Quad Integer(1:w240) -> (0:w239:u64[])
                                n117 = Array Subset(array=w239, index=w238, length=w237) -> (w241:u64[])
                                n118 = Add Array Elements(numeric array=w241) -> (sum=w243:u64)
                                n119 = Divide(x=w243, y=w237) -> (x/y=w242:dbl)
                                }
                                n120 = call <userlib>:"CameraStop.vi"("error in"=w220, "Camera Handle"=w223) -> ("error out"=w218:errorcluster)  [unwired: 1 out]
                                n121 = local write "Intensity Graph"(w214) -> ()
                                n122 = call <userlib>:"ImageDestroy.vi"("error in"=w218, "Data handle"=w217) -> ("error out"=w216:errorcluster)
                                n123 = local write "Waveform Graph"(w200) -> ()
                                n124 = call <userlib>:"FileClose.vi"("error in"=w216, "File Handle"=w222) -> ("error out"=w219:errorcluster)
                                n125 = local write "error out"(w219) -> ()
                                n126 = local read "Filename"() -> (w211:string)
                                n127 = local read "Path"() -> (w213:string)
                                n128 = Format Into String(w198) -> (resulting string=w209:string)  [unwired: 3 in, 1 out]
                                n129 = Format Into String(w199) -> (resulting string=w203:string)  [unwired: 3 in, 1 out]
                                n130 = Concatenate Strings(w213, "\\", w211, "_", w209, "_", w203, "gr") -> (w208:string)
                                n131 = String To Path(string=w208) -> (path=w205:path)
                                n132 = call-poly <vilib>:"Write To Spreadsheet File.vi"("transpose? (no:F)"=TRUE, "format (%.3f)"="%.7f", "1D data"=w200, "file path (dialog if empty)"=w205) -> ()  [unwired: 4 in, 1 out]
                              }
                            }
                          }
                          frame #1 {
                            n133 = Index Array(array=w245, index=w244) -> (element=w249:dbl)
                            n134 = Multiply(x=w249, y=0.00015) -> (x*y=w253:dbl)
                            n135 = Add(x=w253, y="time zero") -> (x+y=w248:dbl)
                            n136 = Absolute Value(x=w248) -> (abs(x)=w252:dbl)
                            n137 = Less?(x=w252, y=49.9) -> (x < y?=w247:bool)
                            n138 = case shown="True" w247 {
                              tunnel: w248 -> [_ w257]
                              frame False {
                              }
                              frame True {
                                n139 = local read "PI Stage Error"() -> (w258:errorcluster)
                                n140 = call "movePI.vi"("PI Stage Error"=w258, "move to position"=w257) -> ("final position"=w256:dbl, "PI Stage Error 2"=w254:errorcluster)
                                n141 = Build Array(w256) -> (w255:dbl[])
                                n142 = local write "PI Stage Error"(w254) -> ()
                                n143 = local write "Position"(w255) -> ()
                              }
                            }
                          }
                          frame #2 {
                            # "Open Actinic Pump shutter"
                            n144 = call "shutter.vi"("error in"=w259, "Shutter Position"=TRUE) -> ("error out"=w260:errorcluster, "Status"=w263:string)  [unwired: 1 in]
                            n145 = local write "error out"(w260) -> ()
                            n146 = local write "Status"(w263) -> ()
                            n147 = Wait (ms)(milliseconds to wait=50) -> ()  [unwired: 1 out]
                          }
                          frame #3 {
                            w282 = 1  # Freerun for example
                            # "Here we save the excited spectrum"
                            n148 = local read "Exposure Time (s)"() -> (w291:dbl)
                            n149 = Bundle(8, 8) -> (w283:cluster{i32, i32})  [unwired: 1 in]
                            n150 = call "ExSubInitSimple.vi"("Intensifier"=FALSE, "Shutter Comp"=w283, "error in (no error)"=w280, "Triggering mode"=w282, "Exposure"=w291, "Camera Handle"=w264) -> ("error out"=w284:errorcluster, "Handles"=w285:cluster{"Camera":u32, "File":u32, "Image":u32})
                            n151 = call "ExSubSnapNStore.vi"("error in (no error)"=w284, "Handle Cluster"=w285) -> ("error out"=w289:errorcluster, "Handle Cluster Out"=w294:T1)
                            n152 = Unbundle(w294) -> ("Image Handle"=w288:u32)  [unwired: 2 out]
                            n153 = Unbundle By Name(w294) -> ("Camera Handle"=w292:u32, "File Handle"=w293:u32, "Image Handle"=w298:u32)
                            n154 = call <userlib>:"ImageGetArrayU16.vi"("error in"=w289, "Z position"=1, "Image Handle"=w288) -> ("error out"=w295:errorcluster, "Array uint 16"=w290:u16[][])  [unwired: 1 out]
                            n155 = Transpose 2D Array(2D array=w290) -> (transposed array=w301:u16[][])
                            n156 = for {
                              N: 1340 -> [_]
                              tunnel: w301 -> [w306] mode=indexing
                              tunnel: [w308] -> w269 mode=indexing
                              n157 = local read "bottom row"() -> (w304:dbl)
                              n158 = local read "width"() -> (w303:dbl)
                              n159 = To Unsigned Quad Integer(1:w306) -> (0:w305:u64[])
                              n160 = Array Subset(array=w305, index=w304, length=w303) -> (w307:u64[])
                              n161 = Add Array Elements(numeric array=w307) -> (sum=w309:u64)
                              n162 = Divide(x=w309, y=w303) -> (x/y=w308:dbl)
                            }
                            n163 = call <userlib>:"CameraStop.vi"("error in"=w295, "Camera Handle"=w292) -> ("error out"=w297:errorcluster)  [unwired: 1 out]
                            n164 = local write "Intensity Graph"(w301) -> ()
                            n165 = call <userlib>:"ImageDestroy.vi"("error in"=w297, "Data handle"=w298) -> ("error out"=w299:errorcluster)
                            n166 = local write "Waveform Graph"(w269) -> ()
                            n167 = call <userlib>:"FileClose.vi"("error in"=w299, "File Handle"=w293) -> ("error out"=w296:errorcluster)
                            n168 = local write "error out"(w296) -> ()
                            n169 = Index Array(array=w266, index=w265) -> (element=w272:dbl)
                            n170 = local read "Filename"() -> (w268:string)
                            n171 = call "tppathcr.vi"("input"=w272) -> ("out"=w273:string)
                            n172 = Format Into String(w264) -> (resulting string=w271:string)  [unwired: 3 in, 1 out]
                            n173 = local read "Path"() -> (w267:string)
                            n174 = Concatenate Strings(w267, "\\", w268, "_", w273, "exc", w271) -> (w277:string)
                            n175 = String To Path(string=w277) -> (path=w275:path)
                            n176 = call-poly <vilib>:"Write To Spreadsheet File.vi"("transpose? (no:F)"=TRUE, "format (%.3f)"="%.7f", "1D data"=w269, "file path (dialog if empty)"=w275) -> ()  [unwired: 4 in, 1 out]
                          }
                          frame #4 {
                            n177 = call "shutter.vi"("error in"=w312, "Shutter Position"=FALSE) -> ("error out"=w313:errorcluster, "Status"=w311:string)  [unwired: 1 in]
                            n178 = local write "error out"(w313) -> ()
                            n179 = local write "Status"(w311) -> ()
                          }
                          frame #5 {
                            n180 = local read "PI Stage Error"() -> (w318:errorcluster)
                            n181 = call "movePI.vi"("PI Stage Error"=w318, "move to position"=10.0) -> ("final position"=w316:dbl, "PI Stage Error 2"=w317:errorcluster)
                            n182 = Build Array(w316) -> (w315:dbl[])
                            n183 = local write "PI Stage Error"(w317) -> ()
                            n184 = local write "Position"(w315) -> ()
                          }
                          frame #6 {
                            n185 = Wait (ms)(milliseconds to wait=300.0) -> ()  [unwired: 1 out]
                          }
                        }
                      }
                    }
                  }
                }
              }
            }
          }
          frame #5 {
            # "move delay stage"
          }
        }
      }
    }
    frame #3 {
      (unwired) "turn off communications with delay stage"
      n186 = local read "PI Stage Error"() -> (w321:errorcluster)
      n187 = call "Close connection if open.vi"("System no."=1, "error in"=w321) -> ("error out"=w320:errorcluster)  [unwired: 16 in, 1 out]
      n188 = local write "PI Stage Error"(w320) -> ()
    }
    frame #4 {
      n189 = call <userlib>:"CameraClose.vi"("error in"=w325, "Camera Handle"=w326) -> ("error out"=w324:errorcluster)
      n190 = call <userlib>:"UninitToolkit.vi"("error in"=w324) -> ("error out"=w323:errorcluster)
      n191 = local write "error out"(w323) -> ()
    }
  }
